vi "未命名 4.vi"() -> ()   [LabVIEW 2017]
panel:
  in  "停止按钮":bool
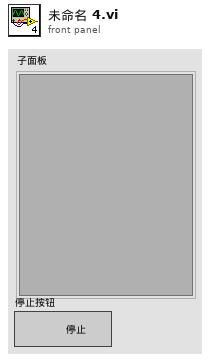
[diagram p1: front panel]
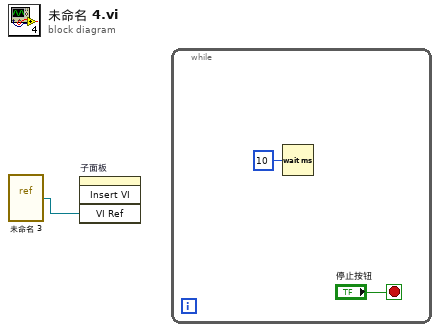
[diagram p0: block diagram]
diagram:
  n1 = vi-ref "未命名 3.vi"() -> (w1:refnum<vi>)
  n2 = invoke on="子面板" class="SubPnl" method="Insert VI"("VI Ref"=w1) -> ()  [unwired: 3 in, 4 out]
  n3 = while {
    stop <- "停止按钮" stop-if-true
    n4 = Wait (ms)(milliseconds to wait=u32 10 ("等待时间（毫秒）")) -> ()  [unwired: 1 out]
  }
